vi "HGCAL_IV.vi"() -> ()   [LabVIEW 2016]
uses:
  <instrlib>/Keithley 24XX/Public/Data/Read (Single Point).vi
  <instrlib>/Keithley 24XX/Keithley 24XX.lvlib
panel:
  in  "Delay Time (s)":dbl=0.1
  in  "Output Base Directory":path=path "Z:/hsinyeh/LabViewToolBox/Data/IV_Curve"
  in  "moduleNumber":string="1"
  in  "fileName":string="test.txt"
  in  "Start":dbl
  in  "End Voltage ( V )":dbl=100.0
  in  "Interval ( V )":dbl=5.0
  in  "Compliance Current (A)":dbl=0.1
  in  "VISA resource name":refnum<visa-resource-name>="COM3"
  in  "Enable Resistance Auto Range (T:Enable)":bool=TRUE
  in  "Enable Current Auto Range (T:Enable)":bool=TRUE
  in  "Enable Voltage Auto Range (T:Enable)":bool=TRUE
  in  "Resistance Manual Range (1.0)":dbl=1.0
  in  "Current Manual Range (1.0)":dbl=1.0
  in  "Voltage Manual Range (1.0)":dbl=1.0
  in  "Serial Configuration":T1={"Baud Rate"=9600, "Parity"=0, "Data Bits"=8, "Stop Bits"=10, "Flow Control"=0} {"Flow Control" items=["None", "XON/XOFF", "RTS/CTS", "XON/XOFF & RTS/CTS", "DTR/DSR", "XON/XOFF & DTR/DSR"]; "Stop Bits" items=["1.0"=10, "1.5"=15, "2.0"=20]; "Data Bits" items=["7"=7, "8"=8]; "Parity" items=["None", "Odd", "Even", "Mark", "Space"]; "Baud Rate" items=["300"=300, "600"=600, "1200"=1200, "2400"=2400, "4800"=4800, "9600"=9600, "19200"=19200]}
  out "IV":cluster{dbl[], dbl[]}(graph)={[5.899888128624298e-05, 5.0004048347473145, 10.000309944152832, 15.00022029876709, 20.000450134277344, 25.00773048400879, 29.997289657592773, 34.98122024536133, 39.98950958251953, 44.97930145263672, 49.967350006103516, 54.97267150878906, 59.959259033203125, 64.95065307617188, 69.95675659179688, 74.95349884033203, 79.95201873779297, 84.97126007080078, 89.97030639648438, 94.9700698852539, 99.9857177734375], [-5.178147147177903e-11, -4.044458865037903e-11, 6.063614887974467e-11, -2.1103530381538782e-11, -1.2681440619832784e-10, -6.122898715821279e-11, -1.026446982965723e-11, -7.520133127325579e-11, 4.0251180860595426e-11, 5.1139849299719486e-11, 2.2053640164054755e-11, -4.2035649266969344e-11, -5.953836035299531e-11, 4.154386903931773e-11, -4.3477641625822017e-11, -3.104800921568951e-12, -7.395824230815862e-11, 6.605579278007312e-11, -8.340572676956981e-11, 6.466382290737371e-11, -5.019033105790882e-11]}
  out "Resistance":sgl=-1992131000000.0
  out "Current":sgl=-5.019033e-11
  out "Voltage":sgl=99.98572
  # "Settings"
  # "IV Curve with keithley 24XX source meter series\nHardware settings with RS-232\nMENU->COMMUNICATION->RS-232->Terminator-><LF>"
  # "Basic Settings (Don't need to change)"
  # "IV Curve"
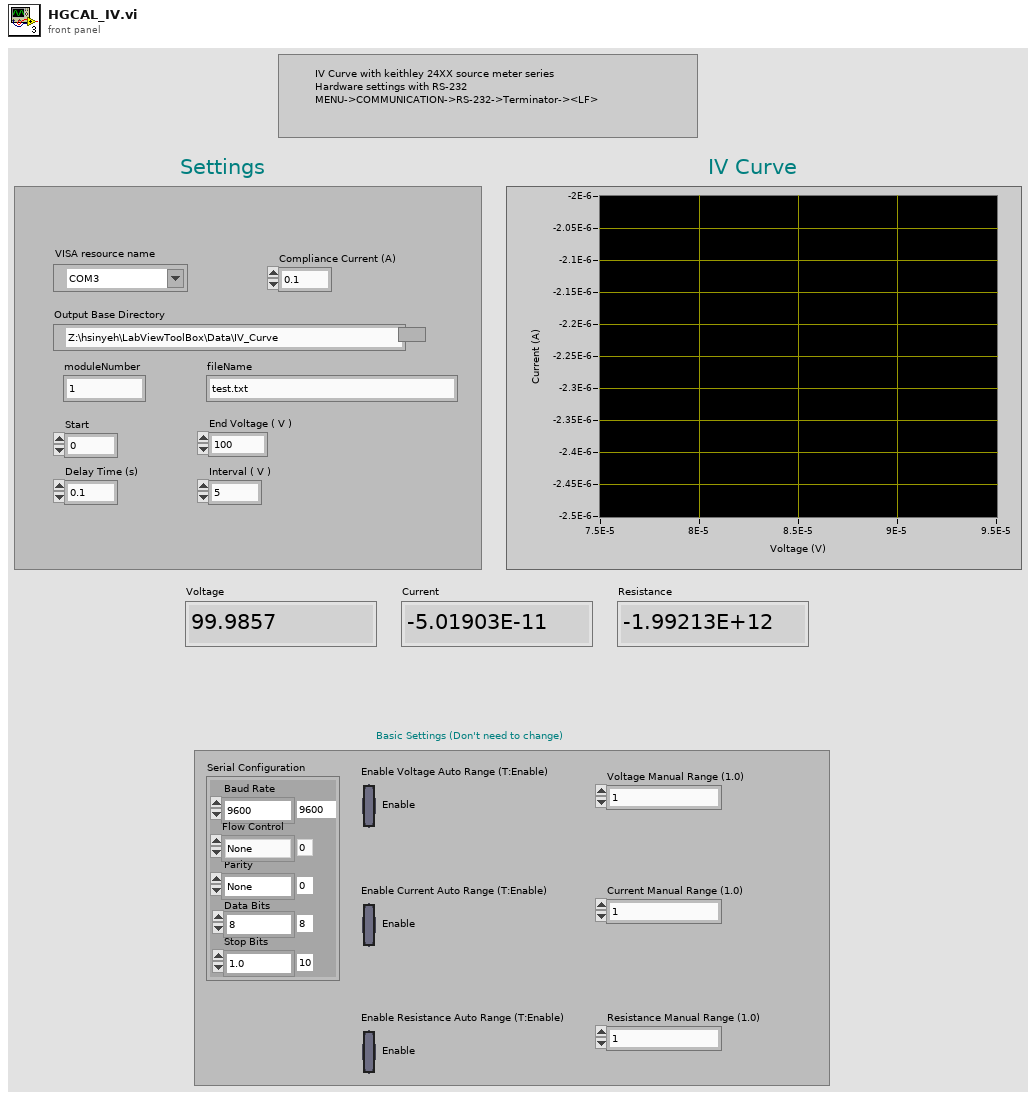
[diagram p1: front panel]
types:
  T1 = cluster{"Baud Rate":u32, "Parity":u16, "Data Bits":u16, "Stop Bits":u16, "Flow Control":u16}
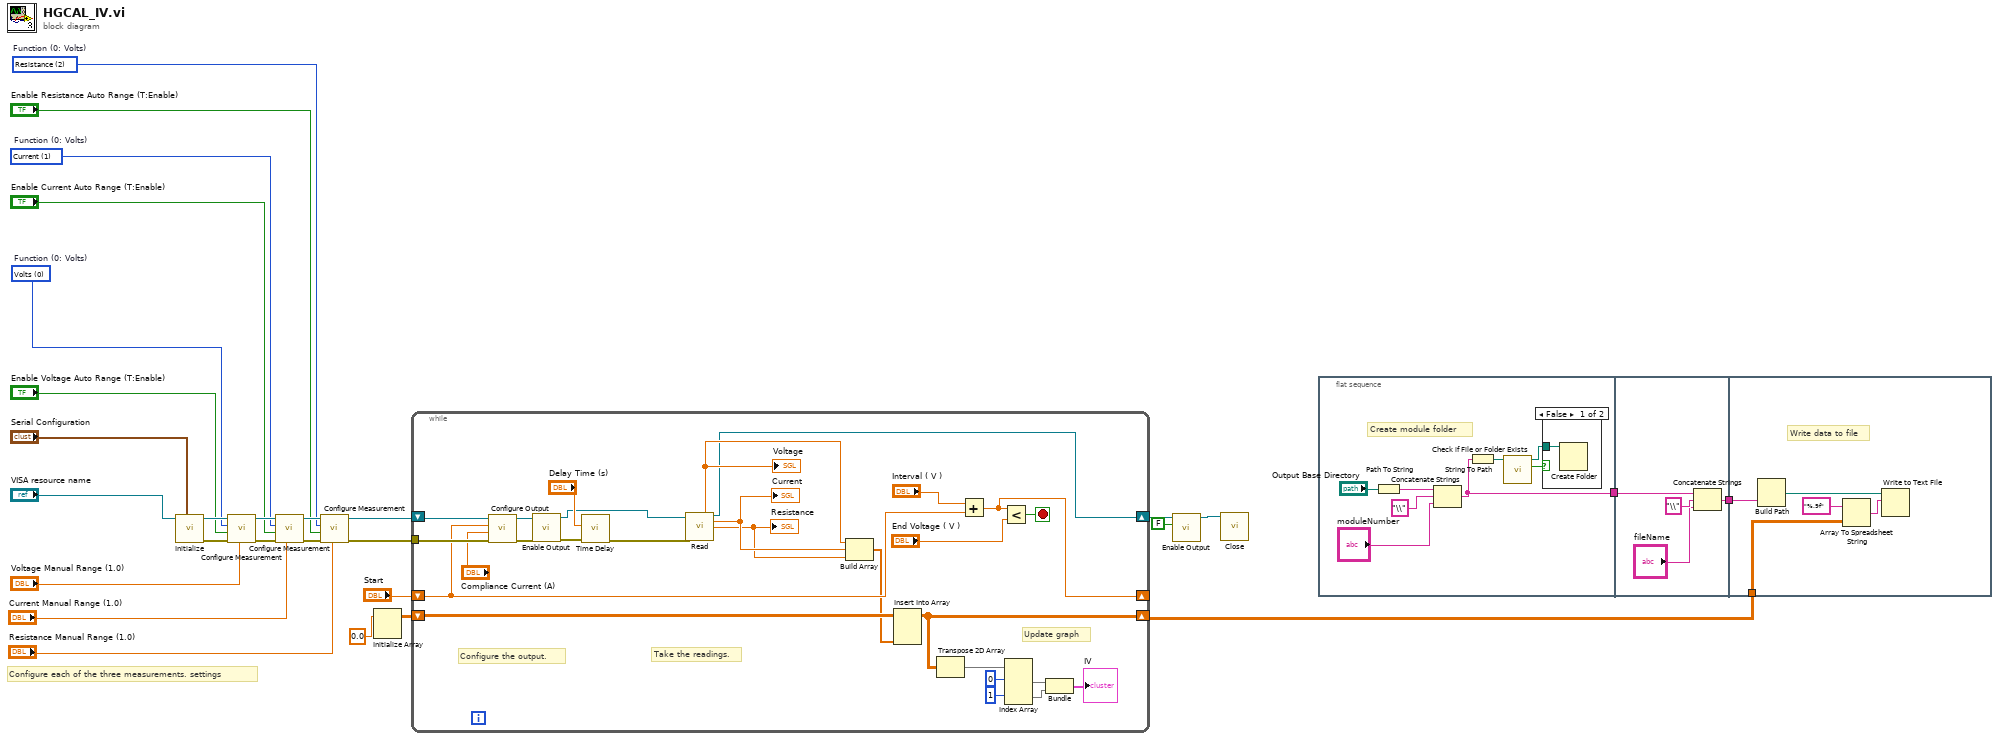
[diagram p0: block diagram]
diagram:
  w18 = u16 2 items=["Volts", "Current", "Resistance"]  # Function (0: Volts)
  w19 = u16 1 items=["Volts", "Current", "Resistance"]  # Function (0: Volts)
  w20 = u16 0 items=["Volts", "Current", "Resistance"]  # Function (0: Volts)
  # "Configure each of the three measurements. settings"
  n1 = call <instrlib>:"Initialize.vi"("Serial Configuration"="Serial Configuration", "VISA resource name"="VISA resource name") -> ("error out"=w25:errorcluster, "VISA resource name out"=w26:refnum<visa-resource-name>)  [unwired: 8 in]
  n2 = call <instrlib>:"Configure Measurement.vi"("Manual Range (1.0)"="Voltage Manual Range (1.0)", "error in (no error)"=w25, "Enable Auto Range (T:Enable)"="Enable Voltage Auto Range (T:Enable)", "Function (0: Volts)"=w20, "VISA resource name"=w26) -> ("error out"=w23:errorcluster, "VISA resource name out"=w24:refnum<visa-resource-name>)  [unwired: 5 in]
  n3 = call <instrlib>:"Configure Measurement.vi"("Manual Range (1.0)"="Current Manual Range (1.0)", "error in (no error)"=w23, "Enable Auto Range (T:Enable)"="Enable Current Auto Range (T:Enable)", "Function (0: Volts)"=w19, "VISA resource name"=w24) -> ("error out"=w22:errorcluster, "VISA resource name out"=w21:refnum<visa-resource-name>)  [unwired: 5 in]
  n4 = call <instrlib>:"Configure Measurement.vi"("Manual Range (1.0)"="Resistance Manual Range (1.0)", "error in (no error)"=w22, "Enable Auto Range (T:Enable)"="Enable Resistance Auto Range (T:Enable)", "Function (0: Volts)"=w18, "VISA resource name"=w21) -> ("error out"=w4:errorcluster, "VISA resource name out"=w5:refnum<visa-resource-name>)  [unwired: 5 in]
  n5 = Initialize Array(0.0 ("element")) -> (w6:dbl[][])  [unwired: 2 in]
  n6 = while {
    tunnel: w4 -> [w54]
    shift-right: [w31] -> _
    shift-left: "Start" -> [w52]
    shift-right: [w48] -> w9
    shift-left: w6 -> [w53]
    shift-right: [w32] -> w3
    shift-left: w5 -> [w55]
    stop <- w29 stop-if-true
    # "Configure the output."
    # "Update graph"
    # "Take the readings."
    n7 = call <instrlib>:"Configure Output.vi"("error in (no error)"=w54, "Compliance  Level (0.1)"="Compliance Current (A)", "Output Level (0)"=w52, "VISA resource name"=w55) -> ("error out"=w37:errorcluster, "VISA resource name out"=w39:refnum<visa-resource-name>)  [unwired: 6 in]
    n8 = call <instrlib>:"Enable Output.vi"("error in (no error)"=w37, "VISA resource name"=w39) -> ("error out"=w36:errorcluster, "VISA resource name out"=w38:refnum<visa-resource-name>)  [unwired: 8 in]
    n9 = call "Time Delay"("error in (no error)"=w36, "Delay Time (s)"="Delay Time (s)") -> ("error out"=w42:errorcluster)  [unwired: 9 in]
    n10 = call-poly <instrlib>:"Read.vi"("VISA resource name"=w38, "error in (no error)"=w42) -> ("Voltage"=w44:sgl, "VISA resource name out"=w32:refnum<visa-resource-name>, "Current"=w45:sgl, "Resistance"=w40:sgl)  [unwired: 7 in, 3 out]
    "Voltage" <- w44
    "Current" <- w45
    "Resistance" <- w40
    n11 = Build Array(w44, w45, w40) -> (w46:sgl[])
    n12 = Insert Into Array(array=w53, new element=w46) -> (w48:dbl[][])  [unwired: 2 in]
    n13 = Transpose 2D Array(2D array=w48) -> (transposed array=w33:dbl[][])
    n14 = Add(x="Interval ( V )", y=w52) -> (x+y=w31:dbl)
    n15 = Less?(x=w31, y="End Voltage ( V )") -> (x < y?=w29:bool)
    n16 = Index Array(array=w33, index (row) #1=0 ("index (row)"), index (row) #2=1 ("index (row)")) -> (element #1=w50:dbl[], element #2=w51:dbl[])  [unwired: 2 in]
    n17 = Bundle(w50, w51) -> (→"IV":cluster{dbl[], dbl[]})  [unwired: 1 in]
  }
  n18 = call <instrlib>:"Enable Output.vi"("Enable Output (T: Enable)"=FALSE, "VISA resource name"=w3) -> ("VISA resource name out"=w1:refnum<visa-resource-name>)  [unwired: 8 in, 1 out]
  n19 = call <instrlib>:"Close.vi"("VISA resource name"=w1) -> ()  [unwired: 10 in, 1 out]
  n20 = flat-sequence {
    tunnel: [w63] -> w10
    tunnel: w10 -> [w68]
    tunnel: [w65] -> w8
    tunnel: w9 -> [w70]
    tunnel: w8 -> [w69]
    frame #0 {
      # "Create module folder"
      n21 = Path To String(path="Output Base Directory") -> (string=w58:string)
      n22 = Concatenate Strings(w58, "\\" ("string"), "moduleNumber") -> (w63:string)
      n23 = String To Path(string=w63) -> (path=w62:path)
      n24 = call <vilib>:"Check if File or Folder Exists.vi"("path"=w62) -> ("file or folder exists?"=w61:bool, "dup path"=w60:path)  [unwired: 8 in, 1 out]
      n25 = case shown="False" w61 {
        tunnel: w60 -> [w64 _]
        frame False {
          n26 = Create Folder(path (use dialog)=w64) -> ()  [unwired: 2 in, 3 out]
        }
        frame True {
        }
      }
    }
    frame #1 {
      n27 = Concatenate Strings(w68, "\\" ("string"), "fileName") -> (w65:string)
    }
    frame #2 {
      # "Write data to file"
      n28 = Build Path(name or relative path=w69) -> (appended path=w73:path)  [unwired: 1 in]
      n29 = Array To Spreadsheet String(array=w70, 3:"%.9f" ("format string")) -> (spreadsheet string=w72:string)  [unwired: 1 in]
      n30 = Write to Text File(file (use dialog)=w73, text=w72) -> ()  [unwired: 2 in, 3 out]
    }
  }
